vi "Heightfield.vi"(4 "Position":cluster{"X":sgl, "Y":sgl, "Z":sgl}, 5 "Alpha":dbl=1.0, 7 "Color Box":u32(colorbox), 8 "error in (no error)":errorcluster, 9 "Size":T1={"Data"=[], "Row Interval"=1.0, "Column Interval"=1.0, "Base Height"=1.0}, 10 "Name":string) -> (0 "error out":errorcluster, 3 "3D Object out":refnum<class "3D Object.lvclass">)   [LabVIEW 2015, in "3D Object.lvclass"]
uses:
  3D Object.lvclass
  <vilib>/picture/3D Picture Control/NI_3D Picture Control.lvlib
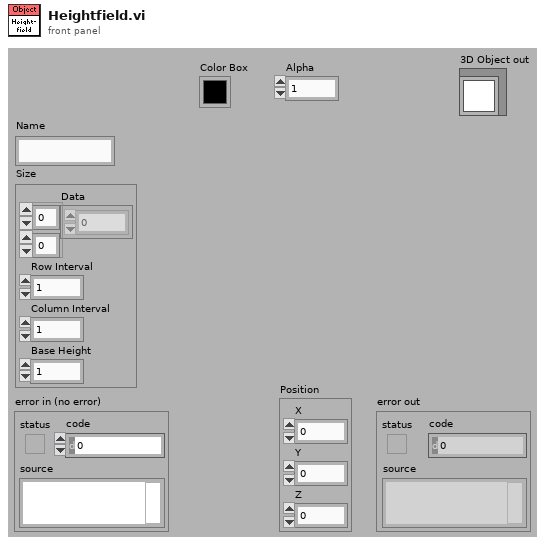
[diagram p1: front panel]
types:
  T1 = cluster{"Data":sgl[][], "Row Interval":sgl, "Column Interval":sgl, "Base Height":sgl}
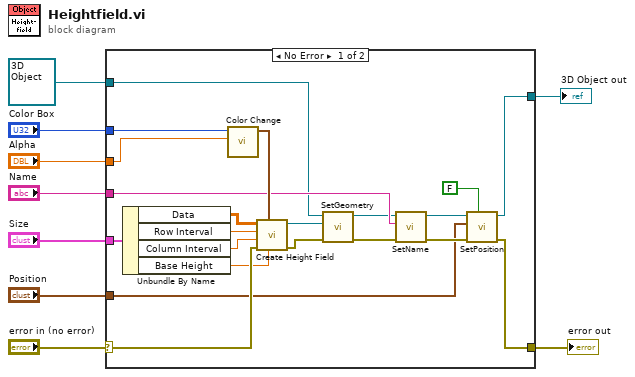
[diagram p0: block diagram]
diagram:
  n1 = case shown="No Error" "error in (no error)" {
    selector: "error in (no error)" -> [w18 w32]
    tunnel: [w25 w32] -> w8
    tunnel: refnum<class "3D Object.lvclass"> refnum ("3D Object in") -> [w17 w31]
    tunnel: [w24 w31] -> w6
    tunnel: "Color Box" -> [w27 _]
    tunnel: "Alpha" -> [w26 _]
    tunnel: "Position" -> [w11 _]
    tunnel: "Name" -> [w23 _]
    tunnel: "Size" -> [w16 _]
    frame No Error {
      n2 = Unbundle By Name(w16) -> ("Data"=w15:sgl[][], "Row Interval"=w14:sgl, "Column Interval"=w13:sgl, "Base Height"=w12:sgl)
      n3 = call <vilib>:"Color Change.vi"("Alpha"=w26, "Color"=w27) -> ("RGBA"=w30:cluster{"R":sgl, "G":sgl, "B":sgl, "A":sgl})  [unwired: 9 out]
      n4 = call <vilib>:"Create Height Field.vi"("Base Height"=w12, "Color"=w30, "error in (no error)"=w18, "Column Interval"=w13, "Row Interval"=w14, "Data"=w15) -> ("error out"=w28:errorcluster, "New Height Field Refnum"=w29:refnum<vi>)  [unwired: 4 in]
      n5 = call "SetGeometry.vi"("error in (no error)"=w28, "Geometry"=w29, "Object in"=w17) -> ("error out"=w21:errorcluster, "Object out"=w22:refnum<class "3D Object.lvclass">)  [unwired: 7 out]
      n6 = call "SetName.vi"("error in (no error)"=w21, "Name"=w23, "3D Object in"=w22) -> ("error out"=w19:errorcluster, "3D Object out"=w20:refnum<class "3D Object.lvclass">)  [unwired: 7 out]
      n7 = call "SetPosition.vi"("Relative?"=FALSE, "error in (no error)"=w19, "Position"=w11, "3D Object in"=w20) -> ("error out"=w25:errorcluster, "3D Object out"=w24:refnum<class "3D Object.lvclass">)  [unwired: 6 in]
    }
    frame Error {
    }
  }
  "error out" <- w8
  "3D Object out" <- w6
